vi "LWXPS_ToString.vi"(3 "LabVIEW error IN":errorcluster, 5 "XPS Reference IN":refnum<k24>) -> (0 "LabVIEW error OUT":errorcluster, 1 "XPS Error String":string, 2 "XPS Reference OUT":refnum<k24>)   [LabVIEW 2014]
uses:
  D:/XPSQ8_LabView_Library/Development/Source/Dll/Newport.XPS.CommandInterface.dll
  Dll/Newport.XPS.CommandInterface.dll
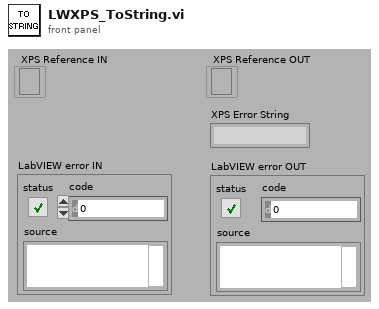
[diagram p1: front panel]
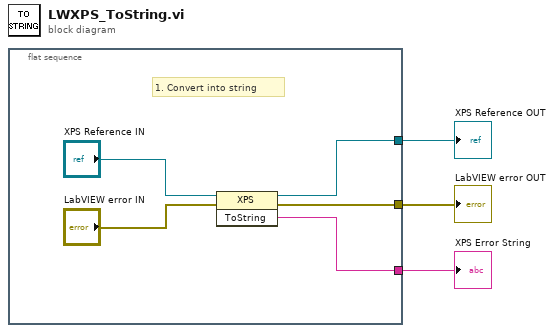
[diagram p0: block diagram]
diagram:
  n1 = flat-sequence {
    tunnel: [w7] -> w3
    tunnel: [w5] -> w2
    tunnel: [w4] -> w1
    frame #0 {
      # "1. Convert into string"
      n2 = invoke class="XPS" method="ToString"(reference="XPS Reference IN", error in="LabVIEW error IN") -> (reference out=w7:refnum<k24>, error out=w5:errorcluster, "ToString"=w4:string)  [unwired: 1 in]
    }
  }
  "XPS Error String" <- w1
  "XPS Reference OUT" <- w3
  "LabVIEW error OUT" <- w2
